vi "要求值表格目录.vi"() -> ()   [LabVIEW 2013]
panel:
  in  "要求值表格目录":path
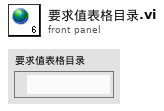
[diagram p1: front panel]
diagram:
